vi "TrajectoryNetwork.vi"(8 "error in (no error)":errorcluster) -> (0 "error out":errorcluster)   [LabVIEW 2023]
uses:
  TrajectoryGlobals.vi
  <vilib>/Rock Robotics/Network Tables/NT Write Number.vi
  <vilib>/Rock Robotics/Network Tables/NT Write Boolean.vi
  <vilib>/Rock Robotics/Network Tables/NT Write Numeric Array.vi
  <vilib>/Rock Robotics/WPI/ThirdParty/JAS_Junk/TrajLib/Trajectory_Library.lvlib
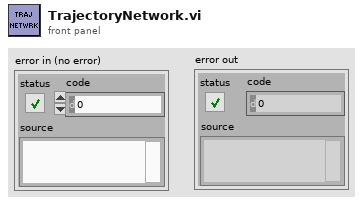
[diagram p1: front panel]
types:
  T1 = typedef "Trajectory_Library.lvlib/POSE2D.ctl" = cluster{"TRANSLATION":T2, "ROTATION":T3}
  T2 = typedef "Trajectory_Library.lvlib/TRANSLATION2D.ctl" = cluster{"X":dbl, "Y":dbl}
  T3 = typedef "Trajectory_Library.lvlib/ROTATION2D.ctl" = cluster{"VALUE":dbl, "COS":dbl, "SIN":dbl}
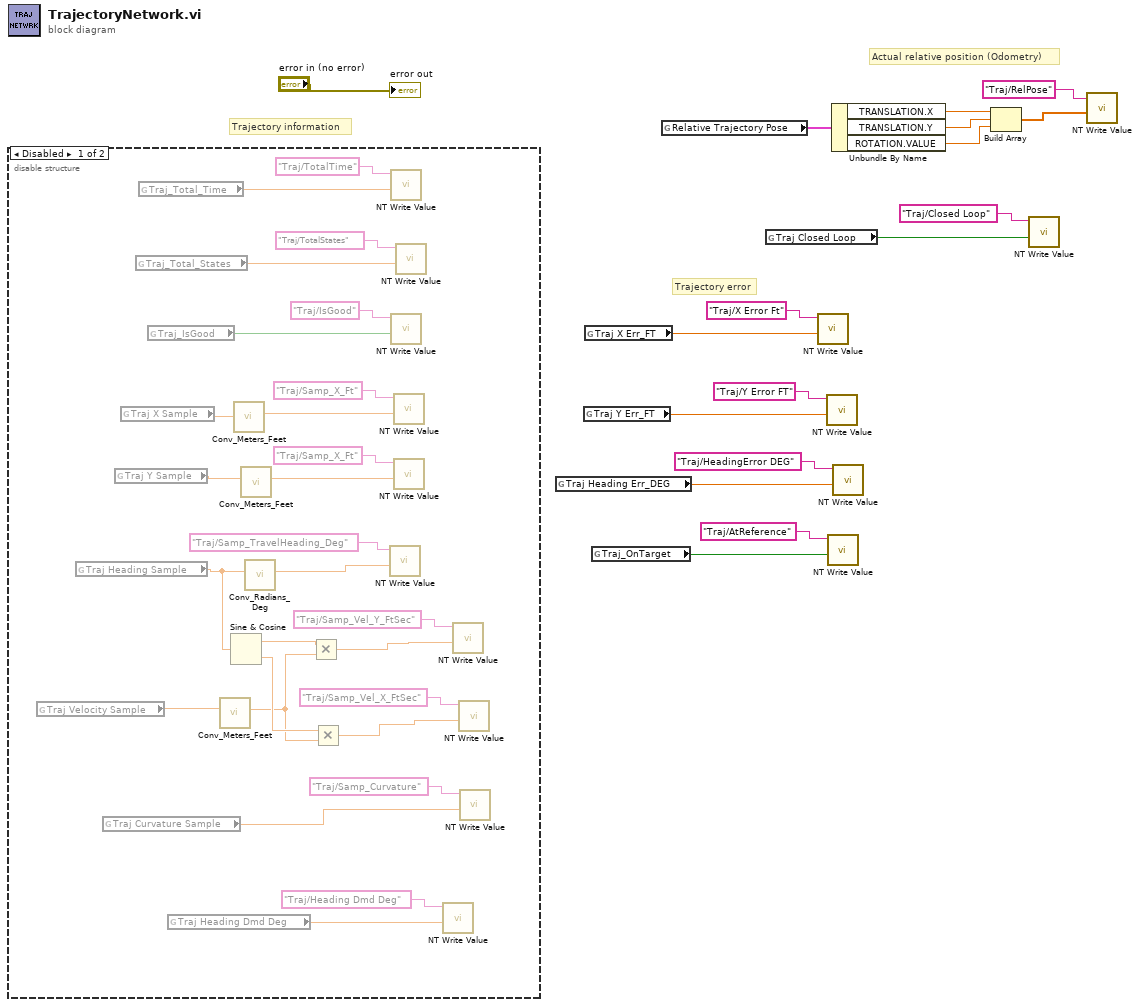
[diagram p0: block diagram]
diagram:
  # "Trajectory information"
  # "Actual relative position (Odometry)"
  # "Trajectory error"
  n1 = disable-structure shown="Disabled" {
    frame Disabled {
      n2 = global read "TrajectoryGlobals.vi" "Traj Velocity Sample"() -> (w27:dbl)
      n3 = global read "TrajectoryGlobals.vi" "Traj Heading Sample"() -> (w28:dbl)
      n4 = global read "TrajectoryGlobals.vi" "Traj Curvature Sample"() -> (w18:dbl)
      n5 = global read "TrajectoryGlobals.vi" "Traj Y Sample"() -> (w31:dbl)
      n6 = global read "TrajectoryGlobals.vi" "Traj X Sample"() -> (w33:dbl)
      n7 = global read "TrajectoryGlobals.vi" "Traj_Total_States"() -> (w38:dbl)
      n8 = global read "TrajectoryGlobals.vi" "Traj_Total_Time"() -> (w37:dbl)
      n9 = global read "TrajectoryGlobals.vi" "Traj_IsGood"() -> (w39:bool)
      n10 = global read "TrajectoryGlobals.vi" "Traj Heading Dmd Deg"() -> (w36:dbl)
      n11 = call <vilib>:"Conv_Meters_Feet.vi"("Meters"=w27) -> ("Feet"=w22:dbl)  [unwired: 10 in]
      n12 = Sine & Cosine(0:w28) -> (1:w24:dbl, 2:w23:dbl)
      n13 = call <vilib>:"Conv_Meters_Feet.vi"("Meters"=w33) -> ("Feet"=w34:dbl)  [unwired: 10 in]
      n14 = call <vilib>:"Conv_Meters_Feet.vi"("Meters"=w31) -> ("Feet"=w32:dbl)  [unwired: 10 in]
      n15 = call <vilib>:"Conv_Radians_Deg.vi"("Radians"=w28) -> ("Degrees"=w29:dbl)  [unwired: 10 in]
      n16 = Multiply(x=w24, y=w22) -> (x*y=w21:dbl)
      n17 = Multiply(x=w23, y=w22) -> (x*y=w20:dbl)
      n18 = call-poly <vilib>:"NT Write Value.vi"("value"=w29, "name"="Traj/Samp_TravelHeading_Deg" ("Name")) -> ()  [unwired: 9 in, 1 out]
      n19 = call-poly <vilib>:"NT Write Value.vi"("value"=w37, "name"="Traj/TotalTime" ("Name")) -> ()  [unwired: 9 in, 1 out]
      n20 = call-poly <vilib>:"NT Write Value.vi"("value"=w39, "name"="Traj/IsGood" ("Name")) -> ()  [unwired: 9 in, 1 out]
      n21 = call-poly <vilib>:"NT Write Value.vi"("value"=w34, "name"="Traj/Samp_X_Ft" ("Name")) -> ()  [unwired: 9 in, 1 out]
      n22 = call-poly <vilib>:"NT Write Value.vi"("value"=w32, "name"="Traj/Samp_X_Ft" ("Name")) -> ()  [unwired: 9 in, 1 out]
      n23 = call-poly <vilib>:"NT Write Value.vi"("value"=w38, "name"="Traj/TotalStates" ("Name")) -> ()  [unwired: 9 in, 1 out]
      n24 = call-poly <vilib>:"NT Write Value.vi"("value"=w36, "name"="Traj/Heading Dmd Deg" ("Name")) -> ()  [unwired: 9 in, 1 out]
      n25 = call-poly <vilib>:"NT Write Value.vi"("value"=w21, "name"="Traj/Samp_Vel_Y_FtSec" ("Name")) -> ()  [unwired: 9 in, 1 out]
      n26 = call-poly <vilib>:"NT Write Value.vi"("value"=w20, "name"="Traj/Samp_Vel_X_FtSec" ("Name")) -> ()  [unwired: 9 in, 1 out]
      n27 = call-poly <vilib>:"NT Write Value.vi"("value"=w18, "name"="Traj/Samp_Curvature" ("Name")) -> ()  [unwired: 9 in, 1 out]
    }
    frame Enabled {
    }
  }
  n28 = global read "TrajectoryGlobals.vi" "Traj Heading Err_DEG"() -> (w4:dbl)
  n29 = global read "TrajectoryGlobals.vi" "Traj Y Err_FT"() -> (w6:dbl)
  n30 = global read "TrajectoryGlobals.vi" "Traj X Err_FT"() -> (w5:dbl)
  n31 = global read "TrajectoryGlobals.vi" "Traj_OnTarget"() -> (w3:bool)
  n32 = global read "TrajectoryGlobals.vi" "Relative Trajectory Pose"() -> (w2:T1)
  n33 = global read "TrajectoryGlobals.vi" "Traj Closed Loop"() -> (w7:bool)
  n34 = call-poly <vilib>:"NT Write Value.vi"("value"=w5, "name"="Traj/X Error Ft" ("Name")) -> ()  [unwired: 9 in, 1 out]
  n35 = call-poly <vilib>:"NT Write Value.vi"("value"=w6, "name"="Traj/Y Error FT" ("Name")) -> ()  [unwired: 9 in, 1 out]
  n36 = call-poly <vilib>:"NT Write Value.vi"("value"=w3, "name"="Traj/AtReference" ("Name")) -> ()  [unwired: 9 in, 1 out]
  n37 = Unbundle By Name(w2) -> ("TRANSLATION.X"=w14:dbl, "TRANSLATION.Y"=w15:dbl, "ROTATION.VALUE"=w16:dbl)
  n38 = call-poly <vilib>:"NT Write Value.vi"("value"=w4, "name"="Traj/HeadingError DEG" ("Name")) -> ()  [unwired: 9 in, 1 out]
  n39 = Build Array(w14, w15, w16) -> (w12:dbl[])
  n40 = call-poly <vilib>:"NT Write Value.vi"("value"=w7, "name"="Traj/Closed Loop" ("Name")) -> ()  [unwired: 9 in, 1 out]
  n41 = call-poly <vilib>:"NT Write Value.vi"("value"=w12, "name"="Traj/RelPose" ("Name")) -> ()  [unwired: 9 in, 1 out]
  "error out" <- "error in (no error)"
